vi "Data Logging Error Replacement.vi"(8 "error in (no error)":errorcluster) -> (0 "error out":errorcluster)   [LabVIEW 2014]
doc: "<B>Copyright</B>: (c) 2015 MHWirth. All rights reserved.\n\nThis subVI replaces known errors with user defined errors."
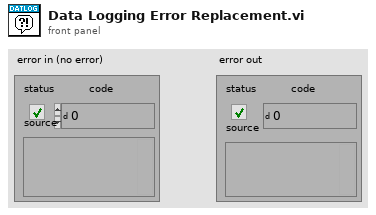
[diagram p1: front panel]
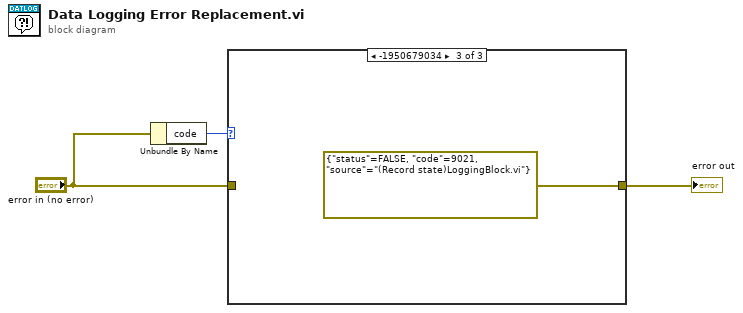
[diagram p0: block diagram]
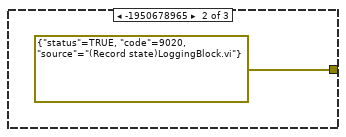
[diagram p3: hidden frame]
diagram:
  n1 = Unbundle By Name("error in (no error)") -> ("code"=w3:i32)
  n2 = case shown="-1950679034" w3 {
    tunnel: [w4 errorcluster {"status"=TRUE, "code"=9020, "source"="(Record state)LoggingBlock.vi"} ("error in (no error)") errorcluster {"status"=FALSE, "code"=9021, "source"="(Record state)LoggingBlock.vi"} ("error in (no error)")] -> w1
    tunnel: "error in (no error)" -> [w4 _ _]
    frame 0, Default {
    }
    frame -1950678965 {
    }
    frame -1950679034 {
    }
  }
  "error out" <- w1
